vi "Prime BSI Set Get Parameter.vi"(0 "Notifier In":refnum<notifier>, 5 "PVCam Actions":T2, 7 "Camera Ref":refnum<k24>, 11 "Error In":errorcluster) -> (4 "Notifier Out":refnum<notifier>, 8 "PVCam Cluster":T1, 15 "Error Out":errorcluster)   [LabVIEW 2020]
uses:
  Prime BSI Type Defs/Prime BSI Actions.ctl
  C:/Users/Public/Documents/Photometrics/PMQI-LabViewSamples BETA/Examples/2020/Dependencies/PVCamNET.dll
  Prime BSI Type Defs/Prime BSI Notifier Element.ctl
  Prime BSI Type Defs/Prime BSI Parameters.ctl
  Prime BSI Type Defs/Prime BSI Parameter List.ctl
  Prime BSI Type Defs/Prime BSI ROI.ctl
  <vilib>/vision/Image Controls.llb/IMAQ Image.ctl
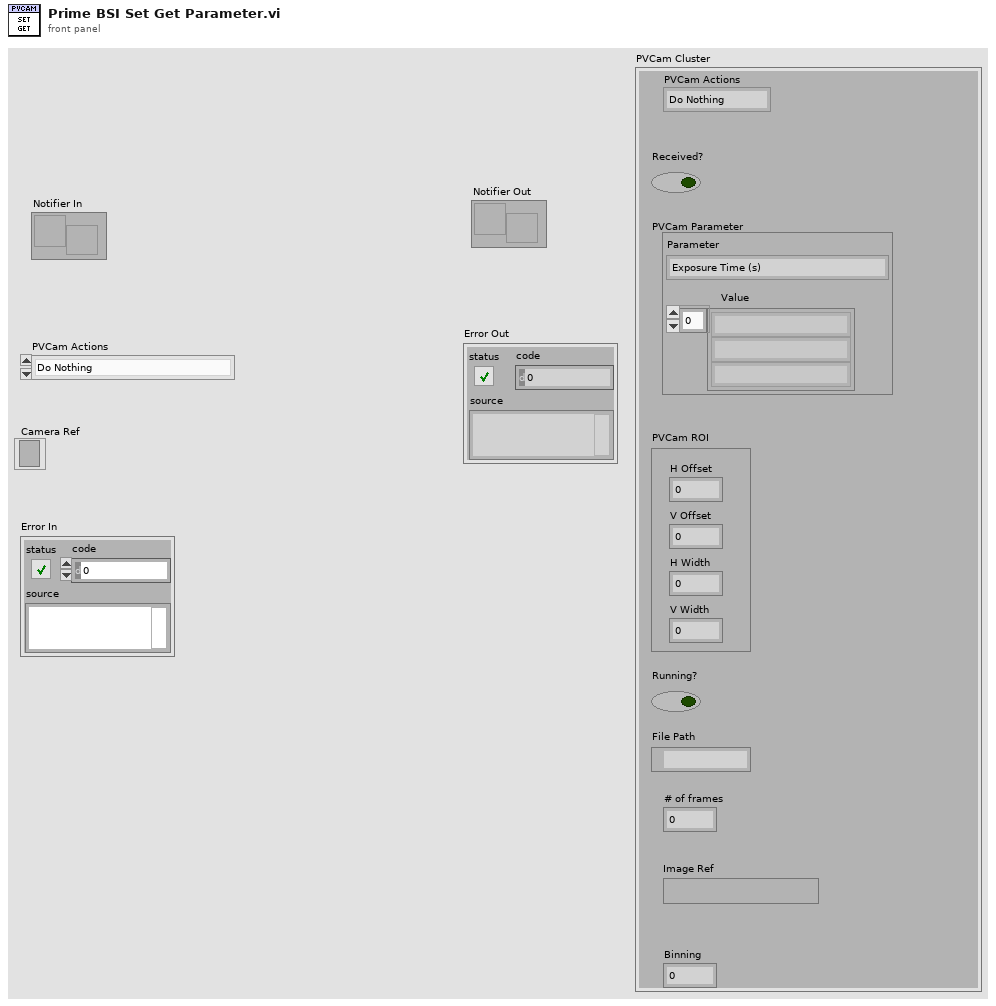
[diagram p1: front panel]
types:
  T1 = typedef "Prime BSI Notifier Element.ctl" = cluster{"PVCam Actions":T2, "Received?":bool, "PVCam Parameter":T3, "PVCam ROI":T5, "Running?":bool, "File Path":path, "# of frames":u32, "Image Ref":T6, "Binning":i32}
  T2 = typedef "Prime BSI Actions.ctl" = enum16{"Do Nothing", "Preview", "Record", "Abort", "Record Settings", "Set Parameter", "Get Parameter", "Set ROI", "Get ROI", "Status", "Quit"}
  T3 = typedef "Prime BSI Parameters.ctl" = cluster{"Parameter":T4, "Value":string[]}
  T4 = typedef "Prime BSI Parameter List.ctl" = enum16{"Exposure Time (s)", "Binning", "Readout Port List", "Available Gain List"}
  T5 = typedef "Prime BSI ROI.ctl" = cluster{"H Offset":i32, "V Offset":i32, "H Width":i32, "V Width":i32}
  T6 = typedef "IMAQ Image.ctl" = refnum<image>
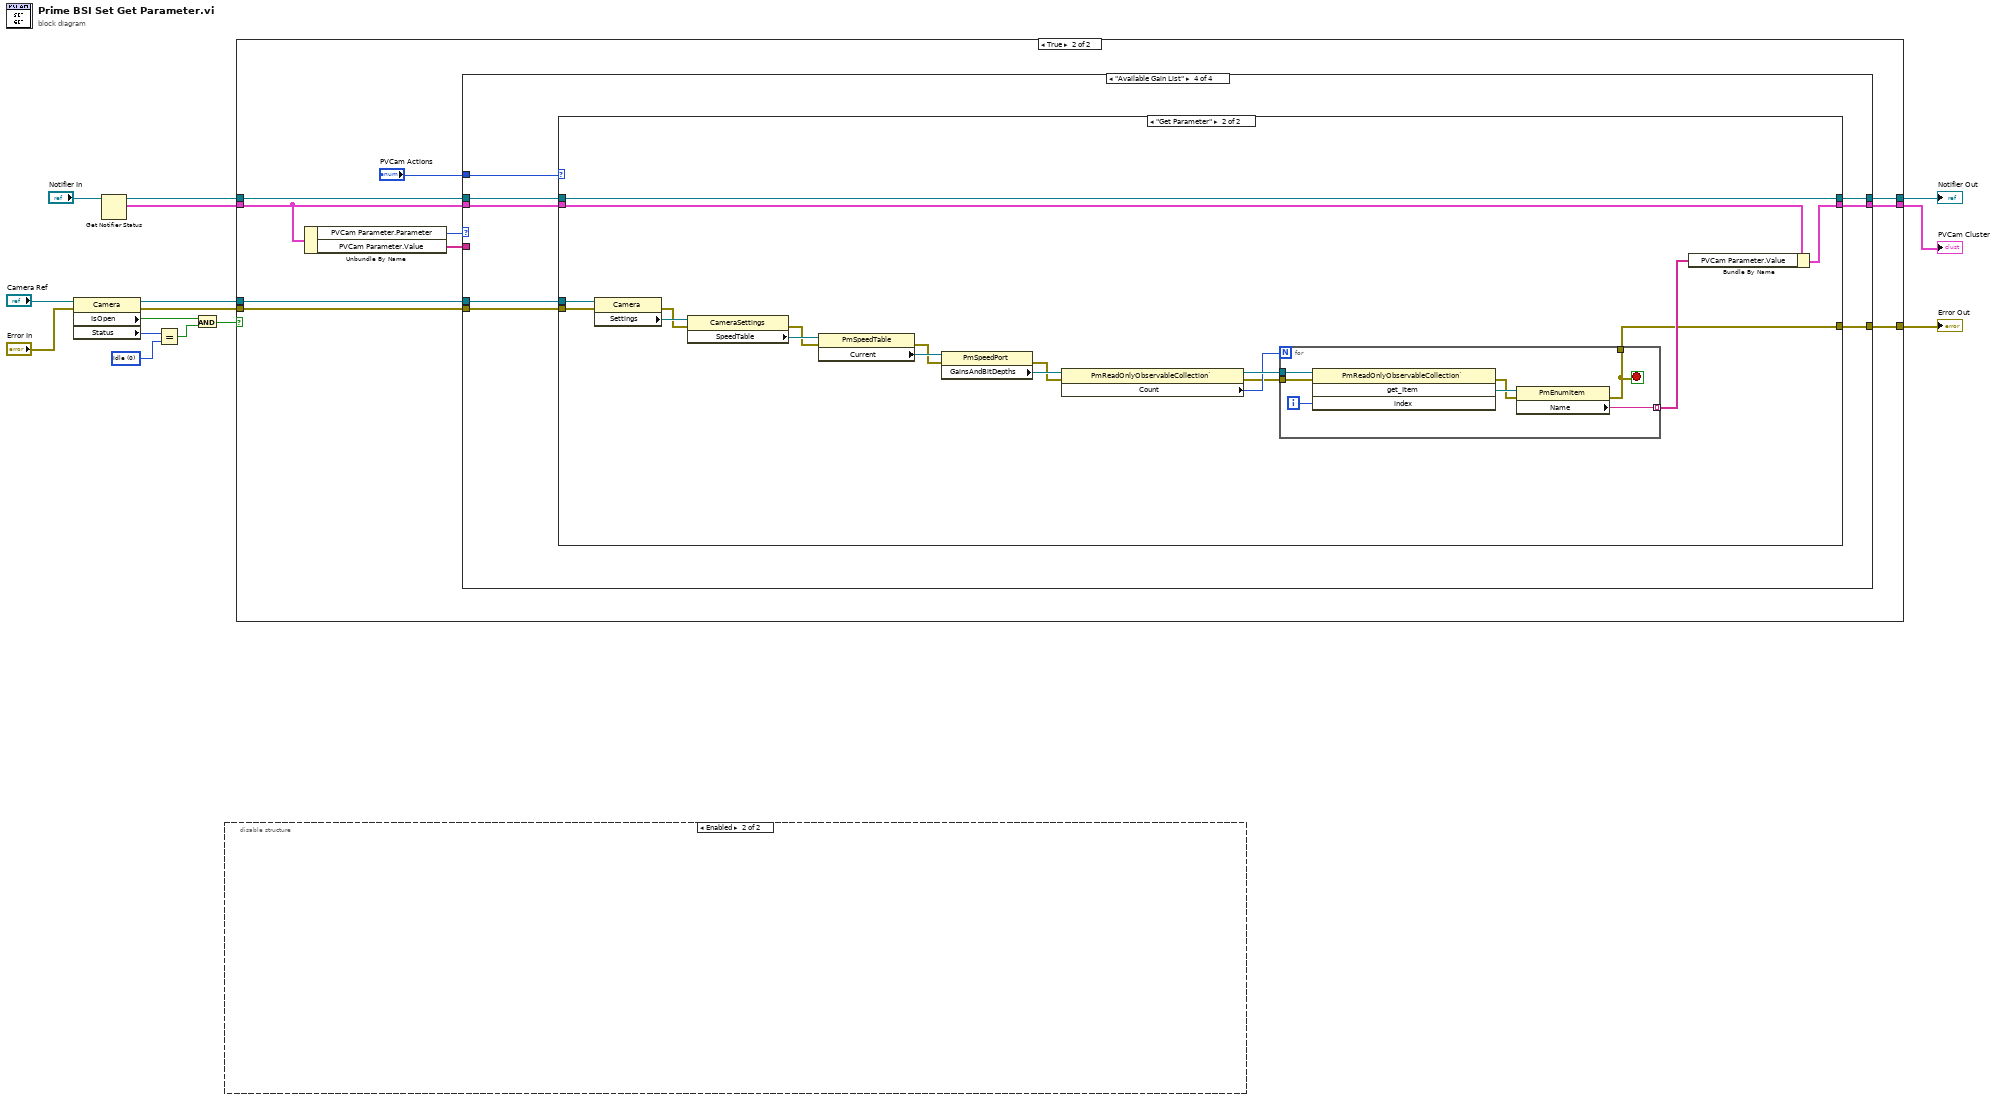
[diagram p0: block diagram]
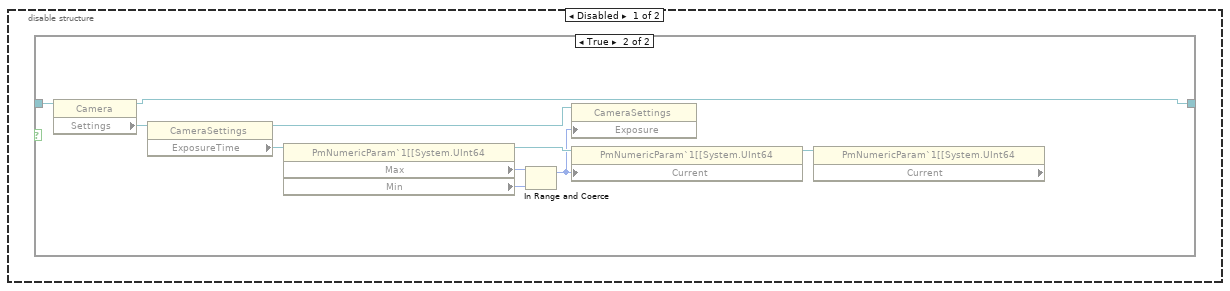
[diagram p2: hidden frame]
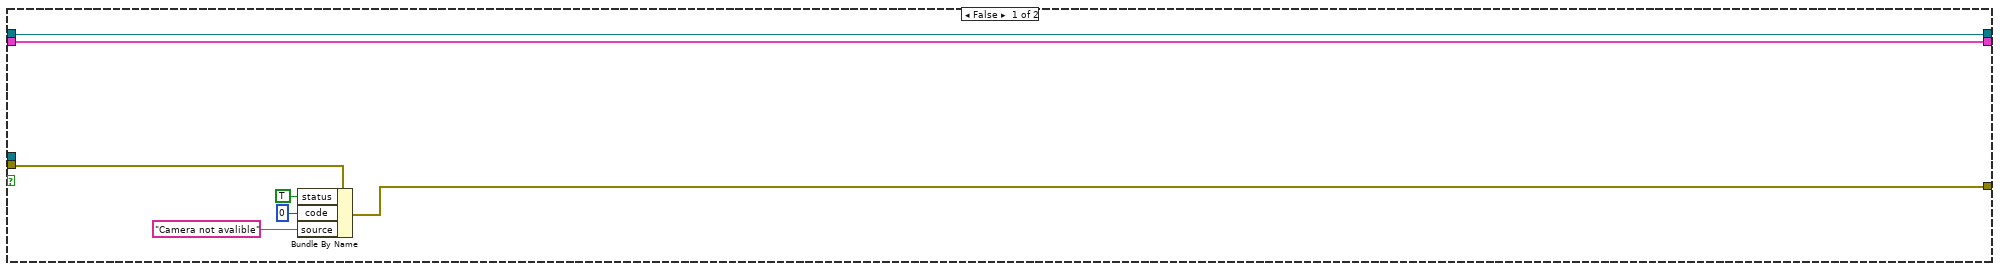
[diagram p4: hidden frame]
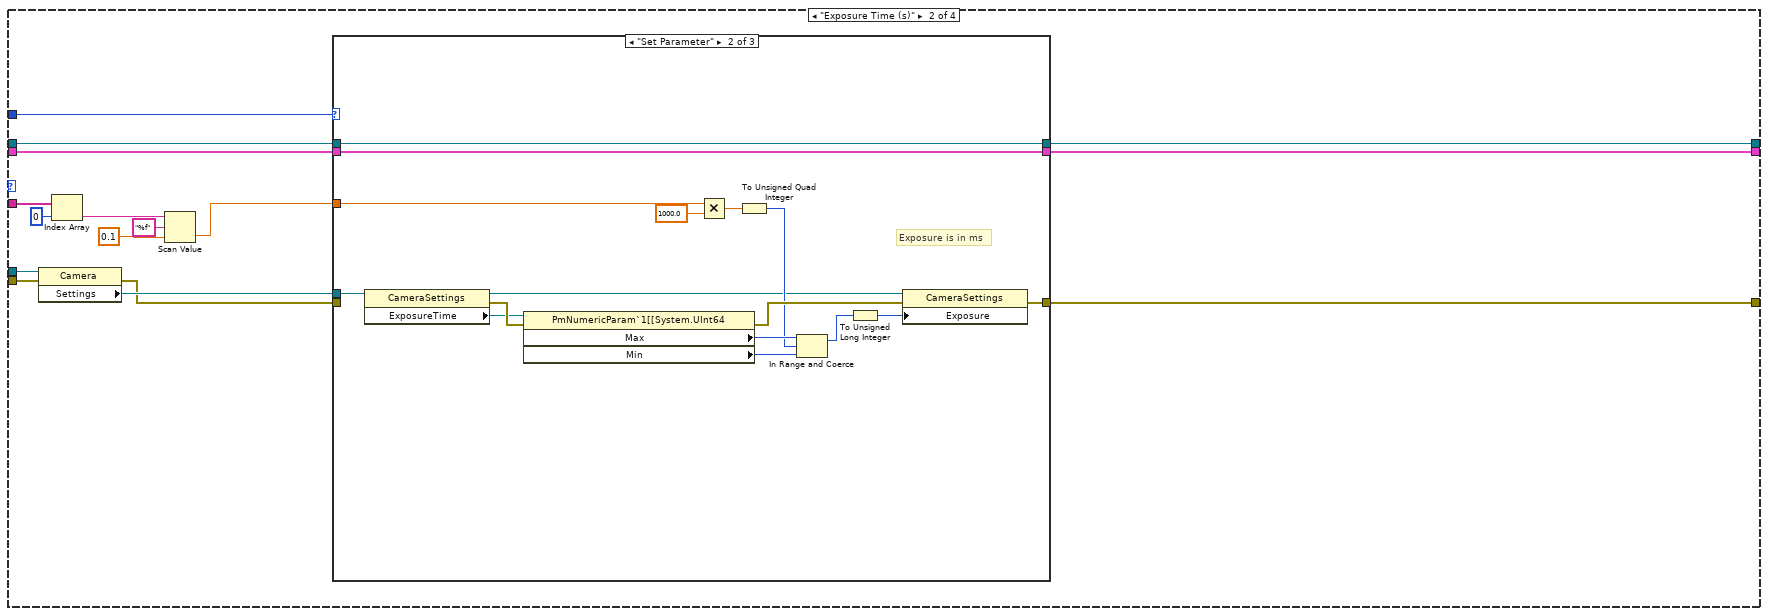
[diagram p6: hidden frame]
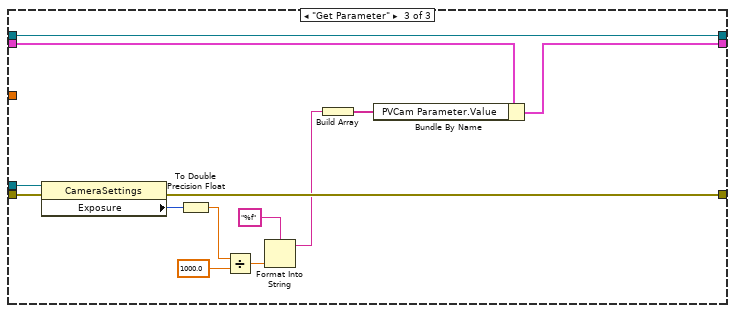
[diagram p8: hidden frame]
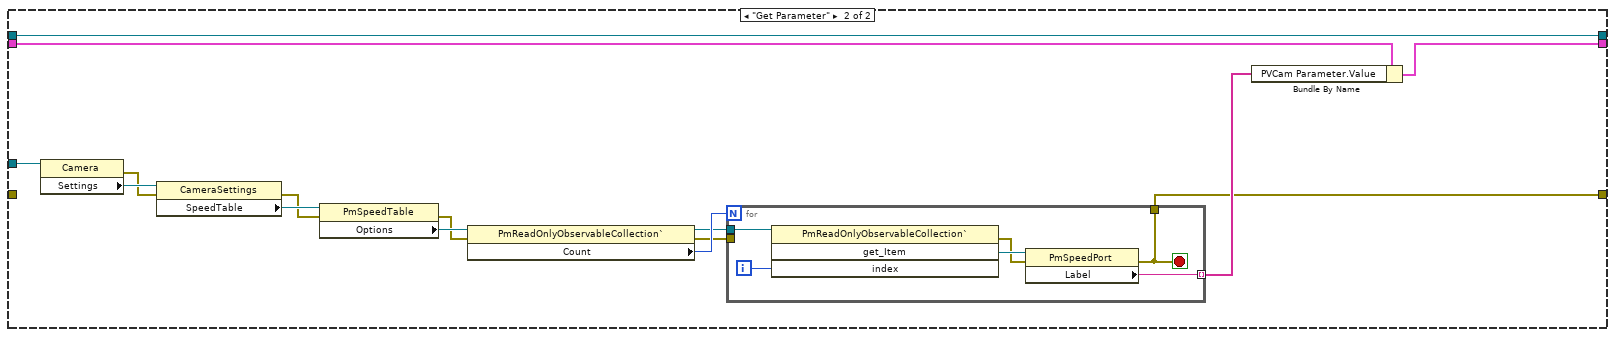
[diagram p10: hidden frame]
diagram:
  w14 = 0 items=["Idle", "Capturing"] ("Status")
  n1 = property class="Camera"(reference="Camera Ref", error in="Error In") -> (reference out=w8:refnum<k24>, error out=w7:errorcluster, "IsOpen"=w13:bool, "Status"=w15:i32)
  n2 = Get Notifier Status(notifier="Notifier In") -> (notifier out=w2:refnum<notifier>, current notification=w1:T1)  [unwired: 1 in, 3 out]
  n3 = Equal?(x=w15, y=w14) -> (x = y?=w12:bool)
  n4 = And(x=w13, y=w12) -> (x .and. y?=w9:bool)
  n5 = disable-structure shown="Enabled" {
    frame Disabled {
      n6 = case shown="True" {
        selector: _ -> [_ _]
        tunnel: _ -> [w16 w26]
        tunnel: [w16 w17] -> _
        frame False {
        }
        frame True {
          n7 = property class="Camera"(reference=w26) -> (reference out=w17:refnum<k24>, "Settings"=w25:refnum<k24>)  [unwired: 1 in, 1 out]
          n8 = property class="CameraSettings"(reference=w25) -> (reference out=w18:refnum<k24>, "ExposureTime"=w19:refnum<k24>)  [unwired: 1 in, 1 out]
          n9 = property class="PmNumericParam`1[[System.UInt64"(reference=w19) -> (reference out=w22:refnum<k24>, "Max"=w24:u64, "Min"=w23:u64)  [unwired: 1 in, 1 out]
          n10 = In Range and Coerce(upper limit=w24, lower limit=w23) -> (coerced(x)=w20:u64)  [unwired: 1 in, 1 out]
          n11 = property class="CameraSettings"(reference=w18, "Exposure"=w20) -> ()  [unwired: 1 in, 2 out]
          n12 = property class="PmNumericParam`1[[System.UInt64"(reference=w22, "Current"=w20) -> (reference out=w21:refnum<k24>)  [unwired: 1 in, 1 out]
          n13 = property class="PmNumericParam`1[[System.UInt64" props=["Current"](reference=w21) -> ()  [unwired: 1 in, 3 out]
        }
      }
    }
    frame Enabled {
    }
  }
  n14 = case shown="True" w9 {
    tunnel: w8 -> [_ w43]
    tunnel: w7 -> [w33 w42]
    tunnel: [w29 w41] -> w6
    tunnel: [w28 w37] -> w5
    tunnel: w2 -> [w28 w35]
    tunnel: [w27 w36] -> w4
    tunnel: w1 -> [w27 w34]
    frame False {
      n15 = Bundle By Name(cluster=w33, "status"=TRUE, "code"=0, "source"="Camera not avalible") -> (w29:errorcluster)
    }
    frame True {
      n16 = Unbundle By Name(w34) -> ("PVCam Parameter.Parameter"=w40:T4, "PVCam Parameter.Value"=w39:string[])
      n17 = case shown="\"Available Gain List\"" w40 {
        tunnel: w43 -> [_ w59 w97 w131]
        tunnel: w42 -> [w45 w58 w95 w132]
        tunnel: w39 -> [_ w52 _ _]
        tunnel: [w45 w62 w96 w127] -> w41
        tunnel: "PVCam Actions" -> [_ w61 w102 w134]
        tunnel: w35 -> [w46 w60 w100 w133]
        tunnel: [w46 w57 w101 w129] -> w37
        tunnel: w34 -> [w44 w54 w99 w130]
        tunnel: [w44 w53 w98 w128] -> w36
        frame Default {
        }
        frame "Exposure Time (s)" {
          n18 = property class="Camera"(reference=w59, error in=w58) -> (error out=w55:errorcluster, "Settings"=w56:refnum<k24>)  [unwired: 1 out]
          n19 = Index Array(array=w52, index=0) -> (element=w50:string)
          n20 = Scan Value(string=w50, format string="%f", default (0 dbl)=0.1) -> (value=w47:dbl)  [unwired: 1 out]
          n21 = case shown="\"Set Parameter\"" w61 {
            tunnel: w47 -> [_ w78 _]
            tunnel: [w65 w72 w93] -> w62
            tunnel: w60 -> [w64 w71 w92]
            tunnel: w56 -> [_ w70 w94]
            tunnel: w55 -> [w65 _ w91]
            tunnel: [w64 w71 w92] -> w57
            tunnel: w54 -> [w63 w66 w87]
            tunnel: [w63 w66 w86] -> w53
            frame Default {
            }
            frame "Set Parameter" {
              # "Exposure is in ms"
              n22 = property class="CameraSettings"(reference=w70) -> (reference out=w69:refnum<k24>, error out=w68:errorcluster, "ExposureTime"=w67:refnum<k24>)  [unwired: 1 in]
              n23 = property class="PmNumericParam`1[[System.UInt64"(reference=w67, error in=w68) -> (error out=w81:errorcluster, "Max"=w80:u64, "Min"=w79:u64)  [unwired: 1 out]
              n24 = Multiply(x=w78, y=1000.0) -> (x*y=w76:dbl)
              n25 = To Unsigned Quad Integer(1:w76) -> (0:w75:u64)
              n26 = In Range and Coerce(upper limit=w80, x=w75, lower limit=w79) -> (coerced(x)=w74:u64)  [unwired: 1 out]
              n27 = To Unsigned Long Integer(number=w74) -> (unsigned 32bit integer=w73:u32)
              n28 = property class="CameraSettings"(reference=w69, error in=w81, "Exposure"=w73) -> (error out=w72:errorcluster)  [unwired: 1 out]
            }
            frame "Get Parameter" {
              n29 = property class="CameraSettings"(reference=w94, error in=w91) -> (error out=w93:errorcluster, "Exposure"=w90:u32)  [unwired: 1 out]
              n30 = To Double Precision Float(number=w90) -> (double precision float=w89:dbl)
              n31 = Divide(x=w89, y=1000.0) -> (x/y=w85:dbl)
              n32 = Format Into String(format string="%f", w85) -> (resulting string=w83:string)  [unwired: 2 in, 1 out]
              n33 = Build Array(w83) -> (w82:string[])
              n34 = Bundle By Name(cluster=w87, "PVCam Parameter.Value"=w82) -> (w86:T1)
            }
          }
        }
        frame "Readout Port List" {
          n35 = case shown="Default" w102 {
            tunnel: [w105 w120] -> w101
            tunnel: w100 -> [w105 w120]
            tunnel: w99 -> [w104 w119]
            tunnel: [w104 w118] -> w98
            tunnel: w97 -> [_ w113]
            tunnel: [w103 w106] -> w96
            tunnel: w95 -> [w103 _]
            frame Default {
            }
            frame "Get Parameter" {
              n36 = property class="Camera"(reference=w113) -> (error out=w116:errorcluster, "Settings"=w117:refnum<k24>)  [unwired: 1 in, 1 out]
              n37 = property class="CameraSettings"(reference=w117, error in=w116) -> (error out=w114:errorcluster, "SpeedTable"=w115:refnum<k24>)  [unwired: 1 out]
              n38 = property class="PmSpeedTable"(reference=w115, error in=w114) -> (error out=w111:errorcluster, "Options"=w112:refnum<k24>)  [unwired: 1 out]
              n39 = property class="PmReadOnlyObservableCollection`"(reference=w112, error in=w111) -> (reference out=w108:refnum<k24>, error out=w109:errorcluster, "Count"=w110:i32)
              n40 = for {
                N: w110 -> [_]
                tunnel: w109 -> [_]
                tunnel: w108 -> [w126]
                tunnel: [w122] -> w107 mode=indexing
                tunnel: [w121] -> w106
                i -> [w125]
                stop <- w121 stop-if-true
                n41 = invoke class="PmReadOnlyObservableCollection`" method="get_Item"(reference=w126, "index"=w125) -> (error out=w123:errorcluster, "get_Item"=w124:refnum<k24>)  [unwired: 2 in, 2 out]
                n42 = property class="PmSpeedPort"(reference=w124, error in=w123) -> (error out=w121:errorcluster, "Label"=w122:string)  [unwired: 1 out]
              }
              n43 = Bundle By Name(cluster=w119, "PVCam Parameter.Value"=w107) -> (w118:T1)
            }
          }
        }
        frame "Available Gain List" {
          n44 = case shown="\"Get Parameter\"" w134 {
            tunnel: w133 -> [w136 w140]
            tunnel: w132 -> [w137 w153]
            tunnel: w131 -> [_ w155]
            tunnel: w130 -> [w135 w142]
            tunnel: [w136 w140] -> w129
            tunnel: [w135 w139] -> w128
            tunnel: [w137 w138] -> w127
            frame Default {
            }
            frame "Get Parameter" {
              n45 = property class="Camera"(reference=w155, error in=w153) -> (error out=w152:errorcluster, "Settings"=w154:refnum<k24>)  [unwired: 1 out]
              n46 = property class="CameraSettings"(reference=w154, error in=w152) -> (error out=w150:errorcluster, "SpeedTable"=w151:refnum<k24>)  [unwired: 1 out]
              n47 = property class="PmSpeedTable"(reference=w151, error in=w150) -> (error out=w148:errorcluster, "Current"=w149:refnum<k24>)  [unwired: 1 out]
              n48 = property class="PmSpeedPort"(reference=w149, error in=w148) -> (error out=w146:errorcluster, "GainsAndBitDepths"=w147:refnum<k24>)  [unwired: 1 out]
              n49 = property class="PmReadOnlyObservableCollection`"(reference=w147, error in=w146) -> (reference out=w145:refnum<k24>, error out=w143:errorcluster, "Count"=w144:i32)
              n50 = for {
                N: w144 -> [_]
                tunnel: w145 -> [w162]
                tunnel: w143 -> [w161]
                tunnel: [w158] -> w141 mode=indexing
                tunnel: [w156] -> w138
                i -> [w160]
                stop <- w156 stop-if-true
                n51 = invoke class="PmReadOnlyObservableCollection`" method="get_Item"(reference=w162, error in=w161, "index"=w160) -> (error out=w157:errorcluster, "get_Item"=w159:refnum<k24>)  [unwired: 1 in, 2 out]
                n52 = property class="PmEnumItem"(reference=w159, error in=w157) -> (error out=w156:errorcluster, "Name"=w158:string)  [unwired: 1 out]
              }
              n53 = Bundle By Name(cluster=w142, "PVCam Parameter.Value"=w141) -> (w139:T1)
            }
          }
        }
      }
    }
  }
  "Error Out" <- w6
  "Notifier Out" <- w5
  "PVCam Cluster" <- w4
